vi "Post-Build Action.vi"(5 "Files Generated by Build":path[](array[path]), 6 "Top Level/Always Included VIs":path[](array[path]), 7 "Destination Path":path, 8 "error in (no error)":errorcluster, 9 "Target Name":string, 10 "Build Specification Name":string, 11 "Project Path":path) -> (0 "error out":errorcluster)   [LabVIEW 2027]
uses:
  Build Automation.lvlib
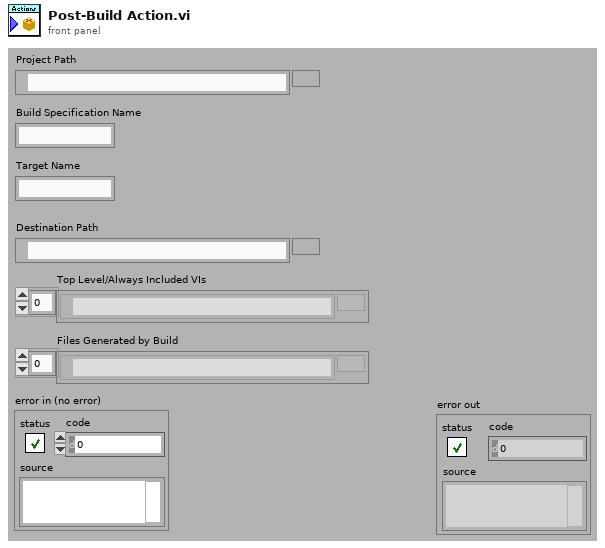
[diagram p1: front panel]
types:
  T1 = cluster{"Status Message":refnum<data-value>, "Progress":refnum<data-value>, "Stop":refnum<data-value>}
  T2 = enum16{"Share clones between instances", "Preallocate clone for each instance"}
  T3 = enum32{"invalid VI type", "Standard VI", "Control VI", "Global VI", "Polymorphic VI", "Configuration VI", "SubSystem", "Facade VI", "Method VI", "Statechart Diagram VI"}
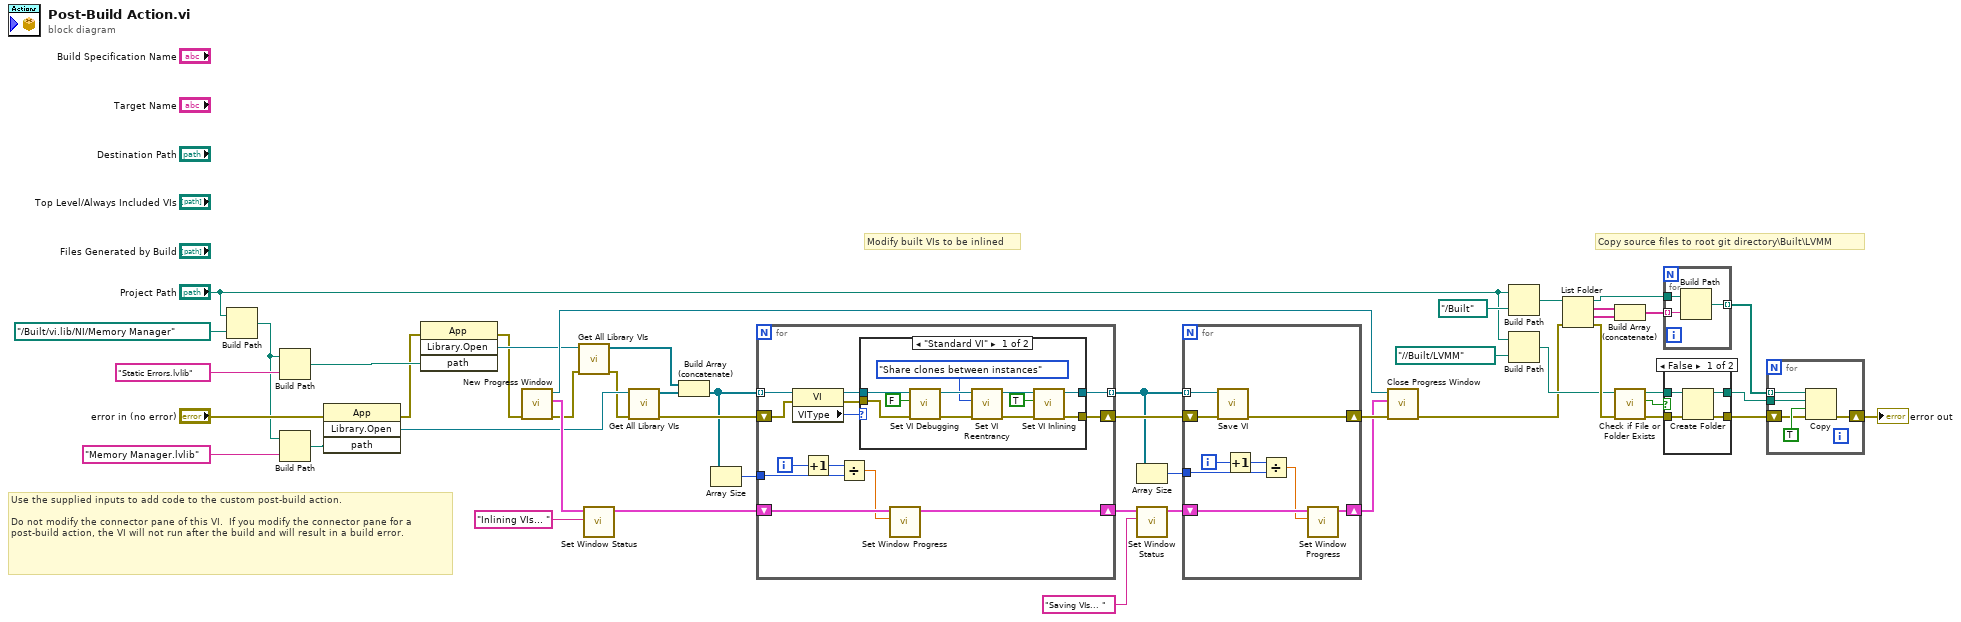
[diagram p0: block diagram]
diagram:
  # "Modify built VIs to be inlined"
  # "Use the supplied inputs to add code to the custom post-build action.\n\nDo not modify the connector pane of this VI.  If you modify the connector pane for a post-build action, the VI will not run after the build and will result in a build error."
  # "Copy source files to root git directory\\Built\\LVMM"
  n1 = Build Path(base path="Project Path", name or relative path=path "../Built/vi.lib/NI/Memory Manager" ("stripped path")) -> (appended path=w15:path)
  n2 = Build Path(base path=w15, name or relative path="Static Errors.lvlib" ("stripped path")) -> (appended path=w13:path)
  n3 = Build Path(base path=w15, name or relative path="Memory Manager.lvlib" ("stripped path")) -> (appended path=w23:path)
  n4 = invoke class="App" method="Library.Open"(error in="error in (no error)", "path"=w23) -> (error out=w8:errorcluster, "Open Library"=w29:refnum<vi>)  [unwired: 2 in, 2 out]
  n5 = invoke class="App" method="Library.Open"(error in=w8, "path"=w13) -> (error out=w7:errorcluster, "Open Library"=w12:refnum<vi>)  [unwired: 2 in, 2 out]
  n6 = call "New Progress Window.vi"("error in (no error)"=w7) -> ("error out"=w6:errorcluster, "DVRs"=w30:T1, "VI refnum"=w34:refnum<vi>)  [unwired: 8 in]
  n7 = call "Get All Library VIs.vi"("error in"=w6, "library ref"=w12) -> ("error out"=w5:errorcluster, "vi refs"=w11:refnum<vi>[])  [unwired: 8 in]
  n8 = call "Set Window Status.vi"("Status Message"="Inlining VIs... " ("data value"), "DVRs in"=w30) -> ("DVRs out"=w35:T1)  [unwired: 8 in, 1 out]
  n9 = call "Get All Library VIs.vi"("error in"=w5, "library ref"=w29) -> ("error out"=w38:errorcluster, "vi refs"=w10:refnum<vi>[])  [unwired: 8 in]
  n10 = Build Array (concatenate)(w11, w10) -> (w9:refnum<vi>[])
  n11 = Array Size(array=w9) -> (size(s)=w36:i32)
  n12 = for {
    tunnel: w9 -> [w54] mode=indexing
    shift-right: [w55] -> w33
    shift-left: w38 -> [w53]
    tunnel: w36 -> [w52]
    shift-right: [w57] -> w32
    shift-left: w35 -> [w59]
    tunnel: [w56] -> w27 mode=indexing
    i -> [w61]
    n13 = property class="VI"(reference=w54, error in=w53) -> (reference out=w51:refnum<vi>, error out=w49:errorcluster, "VIType"=w50:T3)
    n14 = Increment(x=w61) -> (x+1=w60:i32)
    n15 = Divide(x=w60, y=w52) -> (x/y=w58:dbl)
    n16 = case shown="\"Standard VI\"" w50 {
      tunnel: [w65 w73] -> w56
      tunnel: [w62 w74] -> w55
      tunnel: w49 -> [w64 w74]
      tunnel: w51 -> [w63 w73]
      frame "Standard VI" {
        n17 = call "Set VI Debugging.vi"("error in"=w64, "allow debugging"=FALSE ("Allow Debugging"), "vi ref in"=w63) -> ("error out"=w70:errorcluster, "vi ref out"=w71:refnum<vi>)  [unwired: 7 in]
        n18 = call "Set VI Reentrancy.vi"("error in"=w70, "reentrancy type"=T2."Share clones between instances" ("Reentrancy Type"), "vi ref in"=w71) -> ("error out"=w68:errorcluster, "vi ref out"=w69:refnum<vi>)  [unwired: 7 in]
        n19 = call "Set VI Inlining.vi"("error in"=w68, "inline"=TRUE ("Inline VI"), "vi ref in"=w69) -> ("error out"=w62:errorcluster, "vi ref out"=w65:refnum<vi>)  [unwired: 7 in]
      }
      frame Default {
      }
    }
    n20 = call "Set Window Progress.vi"("Progress"=w58, "DVRs in"=w59) -> ("DVRs out"=w57:T1)  [unwired: 8 in, 1 out]
  }
  n21 = Array Size(array=w27) -> (size(s)=w26:i32)
  n22 = call "Set Window Status.vi"("Status Message"="Saving VIs... ", "DVRs in"=w32) -> ("DVRs out"=w28:T1)  [unwired: 8 in, 1 out]
  n23 = for {
    shift-right: [w81] -> w25
    shift-left: w33 -> [w83]
    tunnel: w27 -> [w82] mode=indexing
    shift-right: [w75] -> w24
    shift-left: w28 -> [w77]
    tunnel: w26 -> [w79]
    i -> [w78]
    n24 = call "Save VI.vi"("error in"=w83, "vi ref in"=w82) -> ("error out"=w81:errorcluster)  [unwired: 8 in, 1 out]
    n25 = Increment(x=w78) -> (x+1=w80:i32)
    n26 = Divide(x=w80, y=w79) -> (x/y=w76:dbl)
    n27 = call "Set Window Progress.vi"("Progress"=w76, "DVRs in"=w77) -> ("DVRs out"=w75:T1)  [unwired: 8 in, 1 out]
  }
  n28 = call "Close Progress Window.vi"("error in (no error)"=w25, "DVRs in"=w24, "VI refnum"=w34) -> ("error out"=w22:errorcluster)  [unwired: 8 in]
  n29 = Build Path(base path="Project Path", name or relative path=path "../Built" ("stripped path")) -> (appended path=w40:path)
  n30 = Build Path(base path="Project Path", name or relative path=path "../../Built/LVMM" ("stripped path")) -> (appended path=w39:path)
  n31 = List Folder(path=w40, error in=w22) -> (path out=w44:path, filenames=w4:string[], folder names=w3:string[], error out=w43:errorcluster)  [unwired: 2 in]
  n32 = Build Array (concatenate)(w4, w3) -> (w2:string[])
  n33 = call <vilib>:"Check if File or Folder Exists.vi"("error in (no error)"=w43, "path"=w39) -> ("error out"=w45:errorcluster, "file or folder exists?"=w47:bool, "dup path"=w46:path)  [unwired: 7 in]
  n34 = for {
    tunnel: w2 -> [w85] mode=indexing
    tunnel: w44 -> [w86]
    tunnel: [w84] -> w1 mode=indexing
    n35 = Build Path(base path=w86, name or relative path=w85) -> (appended path=w84:path)
  }
  n36 = case shown="False" w47 {
    tunnel: w46 -> [w90 w92]
    tunnel: w45 -> [w89 w91]
    tunnel: [w88 w92] -> w42
    tunnel: [w87 w91] -> w41
    frame False {
      n37 = Create Folder(path (use dialog)=w90, error in=w89) -> (created path=w88:path, error out=w87:errorcluster)  [unwired: 1 in, 1 out]
    }
    frame True {
    }
  }
  n38 = for {
    tunnel: w1 -> [w94] mode=indexing
    shift-right: [w95] -> w48
    shift-left: w41 -> [w96]
    tunnel: w42 -> [w93]
    n39 = Copy(8:w96, 9:TRUE ("overwrite (F)"), 10:w93, 11:w94) -> (0:w95:errorcluster)  [unwired: 1 in, 2 out]
  }
  "error out" <- w48
